vi "OceanOpticsClose.vi"(8 "error in (no error)":errorcluster, 11 ".NET Refnum in":refnum<k24>) -> (0 "error out":errorcluster)   [LabVIEW 2016]
uses:
  C:/Program Files (x86)/Ocean Optics/OmniDriver/OOI_HOME/NETOmniDriver-NET40.dll
  Program Files (x86)/Ocean Optics/OmniDriver/OOI_HOME/NETOmniDriver-NET40.dll
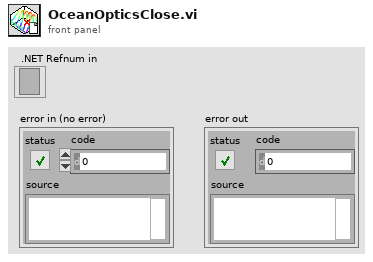
[diagram p1: front panel]
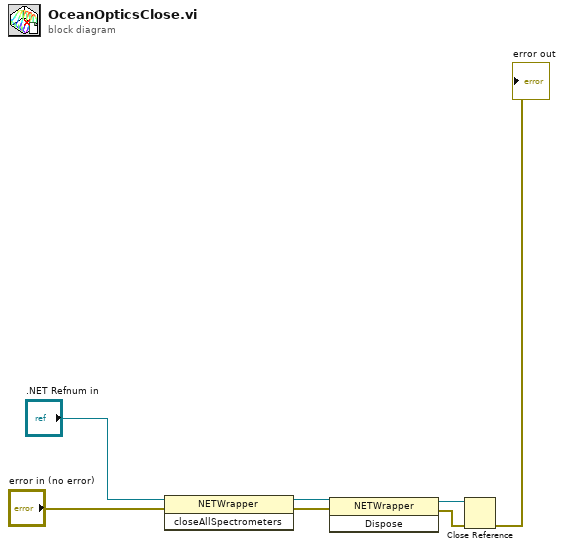
[diagram p0: block diagram]
diagram:
  n1 = invoke class="NETWrapper" method="closeAllSpectrometers"(reference=".NET Refnum in", error in="error in (no error)") -> (reference out=w4:refnum<k24>, error out=w3:errorcluster)  [unwired: 1 in, 1 out]
  n2 = invoke class="NETWrapper" method="Dispose"(reference=w4, error in=w3) -> (reference out=w2:refnum<k24>, error out=w1:errorcluster)  [unwired: 1 in, 1 out]
  n3 = Close Reference(reference=w2, error in (no error)=w1) -> (error out=→"error out":errorcluster)
